vi "AlliGator Phasor Plot Image Cursor Location to Phasor v2.vi"(8 "Error In":errorcluster, 9 "Phasor Plot Size":T1={"H"=512, "V"=512, "Margin"=0.2}, 11 "Coords in":T2) -> (0 "Error Out":errorcluster, 3 "Phasor":T3)   [LabVIEW 2021, in "AlliGator Phasor Plot.lvlib"]
doc: "Converts Phasor Plot Image cursor location to Phasor value."
uses:
  AlliGator Phasor Plot.lvlib
  Phasor/Phasor (g, s).ctl
  <vilib>/Utility/miscctls.llb/LVPoint32TypeDef.ctl
  AlliGator Phasor Plot Size.ctl
  Phasor/Phasor.lvlib
panel:
  # "see the AlliGator License on the block diagram (Ctrl+E or Window:Show Block Diagram)"
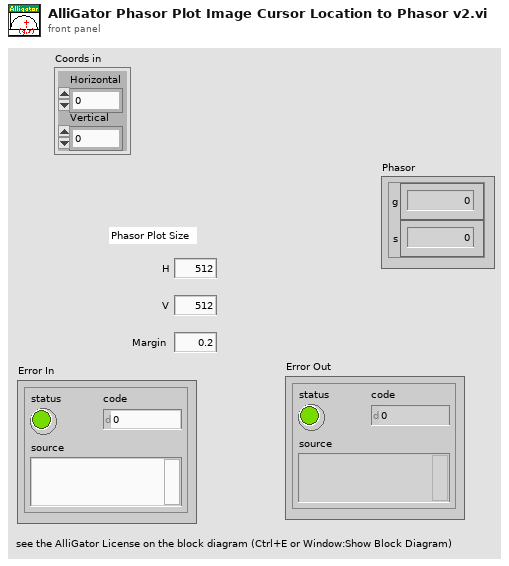
[diagram p1: front panel]
types:
  T1 = typedef "AlliGator Phasor Plot.lvlib/AlliGator Phasor Plot Size.ctl" = cluster{"H":i32, "V":i32, "Margin":dbl}
  T2 = typedef "LVPoint32TypeDef.ctl" = cluster{"Horizontal":i32, "Vertical":i32}
  T3 = typedef "Phasor.lvlib/Phasor (g, s).ctl" = cluster{"g":dbl, "s":dbl}
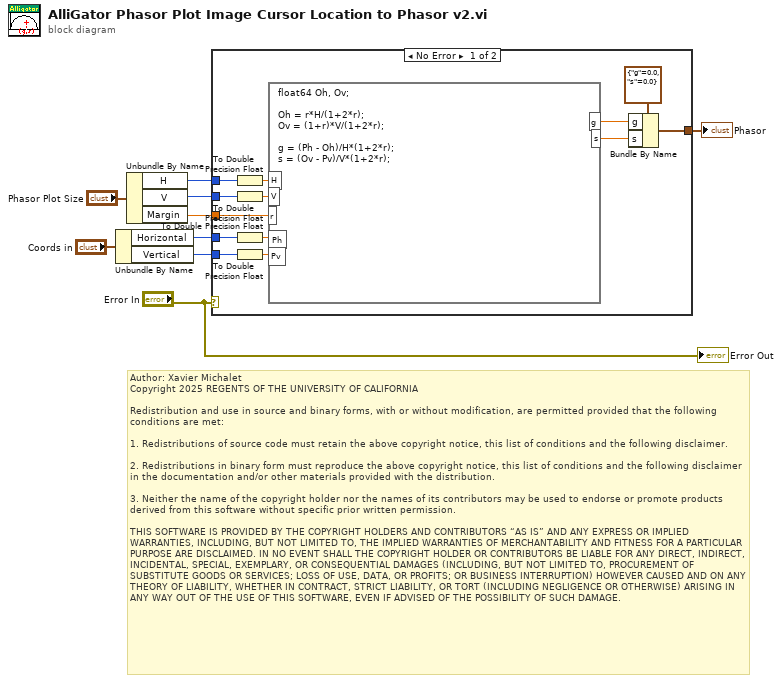
[diagram p0: block diagram]
diagram:
  # "Author: Xavier Michalet\nCopyright 2025 REGENTS OF THE UNIVERSITY OF CALIFORNIA\n\nRedistribution and use in source and binary forms, with or without modification, are permitted provided that the following conditions are met:\n\n1. Redistributions of source code must retain the above copyright notice, this list of conditions and the following disclaimer.\n\n2. Redistributions in binary form must reproduce the above copyright notice, this list of conditions and the following disclaimer in the documentation and/or other materials provided with the distribution.\n\n3. Neither the name of the copyright holder nor the names of its contributors may be used to endorse or promote products derived from this software without specific prior written permission.\n\nTHIS SOFTWARE IS PROVIDED BY THE COPYRIGHT HOLDERS AND CONTRIBUTORS “AS IS” AND ANY EXPRESS OR IMPLIED WARRANTIES, INCLUDING, BUT NOT LIMITED TO, THE IMPLIED WARRANTIES OF MERCHANTABILITY AND FITNESS FOR A PARTICULAR PURPOSE ARE DISCLAIMED. IN NO EVENT SHALL THE COPYRIGHT HOLDER OR CONTRIBUTORS BE LIABLE FOR ANY DIRECT, INDIRECT, INCIDENTAL, SPECIAL, EXEMPLARY, OR CONSEQUENTIAL DAMAGES (INCLUDING, BUT NOT LIMITED TO, PROCUREMENT OF SUBSTITUTE GOODS OR SERVICES; LOSS OF USE, DATA, OR PROFITS; OR BUSINESS INTERRUPTION) HOWEVER CAUSED AND ON ANY THEORY OF LIABILITY, WHETHER IN CONTRACT, STRICT LIABILITY, OR TORT (INCLUDING NEGLIGENCE OR OTHERWISE) ARISING IN ANY WAY OUT OF THE USE OF THIS SOFTWARE, EVEN IF ADVISED OF THE POSSIBILITY OF SUCH DAMAGE."
  n1 = Unbundle By Name("Coords in") -> ("Horizontal"=w4:i32, "Vertical"=w3:i32)
  n2 = Unbundle By Name("Phasor Plot Size") -> ("H"=w6:i32, "V"=w7:i32, "Margin"=w8:dbl)
  n3 = case shown="No Error" "Error In" {
    tunnel: w8 -> [w22 _]
    tunnel: w7 -> [w21 _]
    tunnel: w6 -> [w20 _]
    tunnel: w4 -> [w19 _]
    tunnel: w3 -> [w18 _]
    tunnel: [w15 _] -> w2
    frame No Error {
      n4 = To Double Precision Float(number=w20) -> (double precision float=w13:dbl)
      n5 = To Double Precision Float(number=w21) -> (double precision float=w12:dbl)
      n6 = To Double Precision Float(number=w19) -> (double precision float=w11:dbl)
      n7 = To Double Precision Float(number=w18) -> (double precision float=w10:dbl)
      n8 = formula code="float64 Oh, Ov;\n\nOh = r*H/(1+2*r);\nOv = (1+r)*V/(1+2*r);\n\ng = (Ph - Oh)/H*(1+2*r);\ns = (Ov - Pv)/V*(1+2*r);"("H"=w13, "V"=w12, "r"=w22, "Ph"=w11, "Pv"=w10) -> ("g"=w17:dbl, "s"=w16:dbl)
      n9 = Bundle By Name(cluster=T3 {"g"=0.0, "s"=0.0} ("Phasor"), "g"=w17, "s"=w16) -> (w15:T3)
    }
    frame Error {
    }
  }
  "Phasor" <- w2
  "Error Out" <- "Error In"
